vi "LVClass_WavefrontCorrector Check and Move to Relative Position.vi"(0 "WavefrontCorrector in":refnum<class "WavefrontCorrector.lvclass">, 5 "Sleep after command apply (ms)":i32, 7 "Mirror preferences.Wavefront Corrector State":T2[](array[typedef]), 9 "Position":T1, 11 "error in (no error)":errorcluster) -> (4 "WavefrontCorrector out":refnum<class "WavefrontCorrector.lvclass">, 15 "error out":errorcluster)   [LabVIEW 2020, in "WavefrontCorrector.lvclass"]
uses:
  WavefrontCorrector.lvclass
  Wavefront Corrector states - ONE.ctl
  Wavefront Corrector Position.ctl
  Wavefront Corrector states.ctl
  WavefrontCorrector.lvclass/WavefrontCorrector.ctl
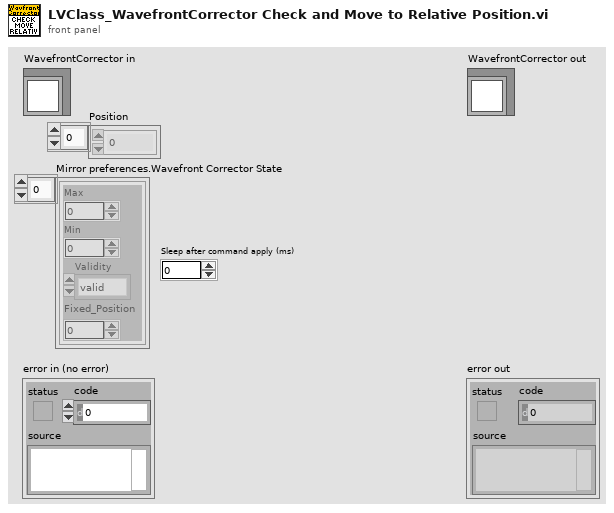
[diagram p1: front panel]
types:
  T1 = typedef "Wavefront Corrector Position.ctl" = sgl[]
  T2 = typedef "Wavefront Corrector states - ONE.ctl" = cluster{"Max":sgl, "Min":sgl, "Validity":enum16{"valid", "fixed", "invalid"}, "Fixed_Position":sgl}
  T3 = typedef "Wavefront Corrector states.ctl" = cluster{"Sleep after command apply_ms":i32, "Wavefront Corrector State":T2[], "WavefrontCorrectorOffsetState":sgl[]}
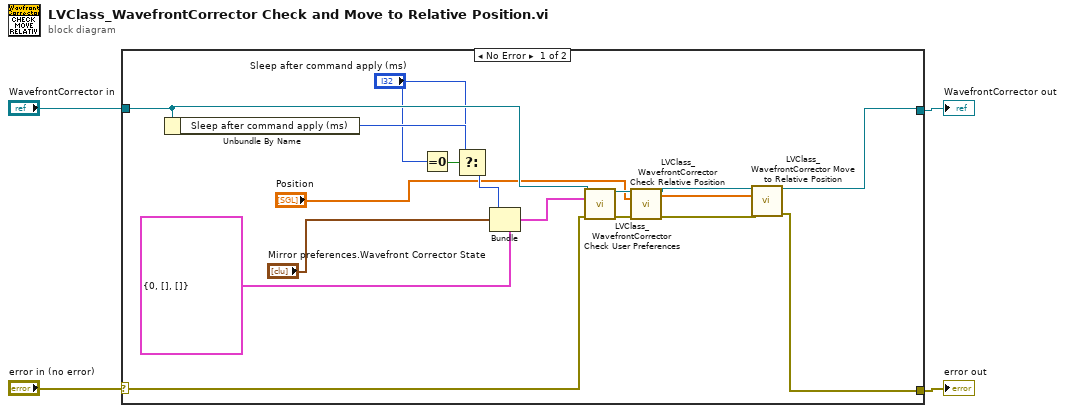
[diagram p0: block diagram]
diagram:
  n1 = case shown="No Error" "error in (no error)" {
    selector: "error in (no error)" -> [w16 w23]
    tunnel: [w18 w23] -> w1
    tunnel: [w20 w22] -> w2
    tunnel: "WavefrontCorrector in" -> [w12 w22]
    frame No Error {
      n2 = Unbundle By Name(w12) -> ("Sleep after command apply (ms)"=w10:i32)
      n3 = Equal To 0?(x="Sleep after command apply (ms)") -> (x = 0?=w11:bool)
      n4 = Select(t=w10, s=w11, f="Sleep after command apply (ms)") -> (s? t:f=w9:i32)
      n5 = Bundle(cluster=T3 {"Sleep after command apply_ms"=0, "Wavefront Corrector State"=[], "WavefrontCorrectorOffsetState"=[]} ("Mirror preferences"), "Sleep after command apply_ms"=w9, "Wavefront Corrector State"="Mirror preferences.Wavefront Corrector State") -> (w14:T3)  [unwired: 1 in]
      n6 = call "LVClass_WavefrontCorrector Check User Preferences.vi"("WavefrontCorrector in"=w12, "Mirror preferences"=w14, "error in (no error)"=w16) -> ("WavefrontCorrector out"=w13:refnum<class "WavefrontCorrector.lvclass">, "error out"=w15:errorcluster)  [unwired: 11 in]
      n7 = call "LVClass_WavefrontCorrector Check Relative Position.vi"("WavefrontCorrector in"=w13, "Relative Positions"="Position", "error in (no error)"=w15) -> ("WavefrontCorrector out"=w21:refnum<class "WavefrontCorrector.lvclass">, "Relative Positions OUT"=w17:T1, "error out"=w19:errorcluster)  [unwired: 10 in]
      n8 = call "LVClass_WavefrontCorrector Move to Relative Position.vi"("WavefrontCorrector in"=w21, "Wavefront Relative Position"=w17, "error in (no error)"=w19) -> ("WavefrontCorrector out"=w20:refnum<class "WavefrontCorrector.lvclass">, "error out"=w18:errorcluster)  [unwired: 11 in]
    }
    frame Error {
    }
  }
  "error out" <- w1
  "WavefrontCorrector out" <- w2
